vi "Teleop[Conflict].vi"(10 "Match Info":T3={"Autonomous Elapsed Seconds"=0.0, "TeleOp Elapsed Seconds"=0.0, "Disabled Elapsed Seconds"=0.0, "Visited Autonomous"=FALSE, "Visited TeleOp"=FALSE, "Visited Disabled"=FALSE, "Autonomous Settings"={"Autonomous Style"=enum."Independent", "VI Refnum"=refnum}}, 11 "Call Context":T4) -> ()   [LabVIEW 2019]
doc: "This VI is called for each TeleOp packet received from the DS where the robot is not disabled. It is often used to read from the joysticks and update I/O or to update setpoints for timed control loops. It should complete and return within 20 milliseconds or it may miss DS packets."
uses:
  <vilib>/Rock Robotics/WPI/DriverStation/WPI_DriverStationDerivedRobotMode.ctl
  <vilib>/Rock Robotics/WPI/DriverStation/WPI_DriverStationMatch Info.ctl
  <vilib>/Rock Robotics/WPI/ThirdParty/Phoenix-LabVIEW/Motor Controller/Controls/CTRE_Phoenix_MotorControl_ControlMode.ctl
  <vilib>/Rock Robotics/WPI/Utilities/WPI_GetSetVariantRefNum.vi
  <vilib>/Rock Robotics/WPI/Joystick/WPI_JoystickArcadeMapping.vi
  Toolbox/Piston/Piston Toggle.vi
  <vilib>/Rock Robotics/WPI/Solenoid/WPI_SolenoidSetEnum.vi
  <vilib>/Rock Robotics/WPI/ThirdParty/Phoenix-LabVIEW/Motor Controller/Get/CTRE_Phoenix_MotorController_GetSupplyAndStatorCurrent_Enhanced.vi
  <vilib>/Rock Robotics/Network Tables/NT Read Number.vi
  <vilib>/addons/control/pid/pid.llb/PID (DBL).vi
  <vilib>/addons/control/pid/NI_PID_pid.lvlib
panel:
  in  "Shooter Power":dbl=1.0
  in  "Auto Mode":enum16{"Manual", "Old Auto", "New Auto"}(ring)
  in  "Magazine Recovery Power":dbl=0.5
  in  "Magazine Intake power":dbl=0.25
  in  "Idle flywheel power":dbl
  in  "Flywheel power":dbl
  in  "Magazine power":dbl
  in  "Intake power":dbl=0.7
  out "Shooter Motor Current":T1(graph)
  out "tx":dbl
  in  "PID gains":T2={"proportional gain (Kc)"=0.05, "integral time (Ti, min)"=0.0, "derivative time (Td, min)"=0.0} {"derivative time (Td, min)" format="%.3g"; "integral time (Ti, min)" format="%.3e"; "proportional gain (Kc)" format="%.3g"}
  in  "Winch Power":dbl=1.0
  in  "Intake Power":dbl=1.0
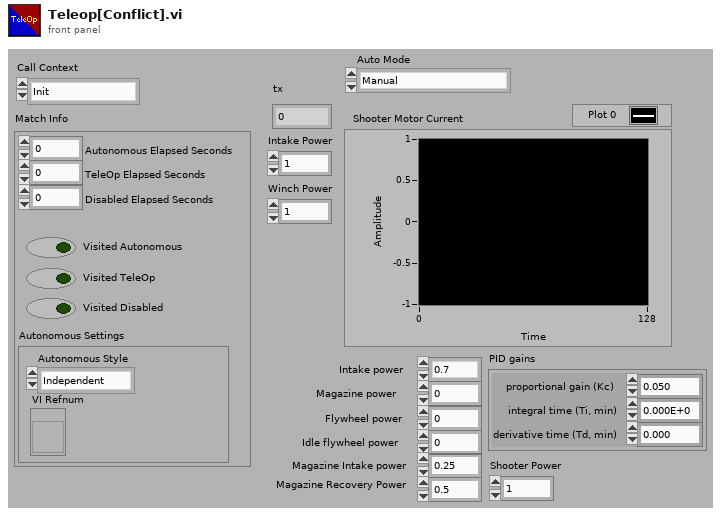
[diagram p1: front panel]
types:
  T1 = cluster{"Supply Current":dbl, "Stator Current":dbl}
  T2 = cluster{"proportional gain (Kc)":dbl, "integral time (Ti, min)":dbl, "derivative time (Td, min)":dbl}
  T3 = typedef "WPI_DriverStationMatch Info.ctl" = cluster{"Autonomous Elapsed Seconds":dbl, "TeleOp Elapsed Seconds":dbl, "Disabled Elapsed Seconds":dbl, "Visited Autonomous":bool, "Visited TeleOp":bool, "Visited Disabled":bool, "Autonomous Settings":cluster{"Autonomous Style":enum16{"Iterative", "Independent"}, "VI Refnum":refnum<vi>}}
  T4 = typedef "WPI_DriverStationDerivedRobotMode.ctl" = enum16{"Init", "Execute", "Stop"}
  T5 = cluster{"Intake In":bool, "Intake Out":bool, "Magazine In":bool, "Magazine Out":bool, "Winch In":bool, "Winch Out":bool, "Climber Hold":bool, "Intake Pistons":bool, "Shooter Hold":bool, "None":bool, "Power Toggle":bool, "Auto Target":bool}
  T6 = typedef "CTRE_Phoenix_MotorControl_ControlMode.ctl" = u16
  T7 = typedef "WPI_JoystickDevRef.ctl" = cluster{"Device":T8}
  T8 = typedef "WPI_JoystickDeviceEnum.ctl" = enum16{"USB 0", "USB 1", "USB 2", "USB 3", "USB 4", "USB 5"}
  T9 = typedef "WPI_SolenoidValue.ctl" = enum16{"Off", "On", "Forward", "Reverse"}
  T10 = typedef "WPI_SolenoidDevRef.ctl" = cluster{"DevStatus":errorcluster, "Pneumatics Control Module":u8, "Forward Solenoid Channel":T11, "Reverse Solenoid Channel":T11}
  T11 = typedef "WPI_SolenoidChannel.ctl" = enum8{"Solenoid 0", "Solenoid 1", "Solenoid 2", "Solenoid 3", "Solenoid 4", "Solenoid 5", "Solenoid 6", "Solenoid 7", "Invalid"}
  T12 = typedef "WPI_DigitalInputDevRef.ctl" = cluster{"DevStatus":errorcluster, "DIO Channel":T13}
  T13 = typedef "FPGA_DIOChannel.ctl" = enum8{"DIO 0", "DIO 1", "DIO 2", "DIO 3", "DIO 4", "DIO 5", "DIO 6", "DIO 7", "DIO 8", "DIO 9", "DIO MXP 0", "DIO MXP 1", "DIO MXP 2", "DIO MXP 3", "DIO MXP 4", "DIO MXP 5", "DIO MXP 6", "DIO MXP 7", "DIO MXP 8", "DIO MXP 9", "DIO MXP 10", "DIO MXP 11", "DIO MXP 12", "DIO MXP 13", "DIO MXP 14", "DIO MXP 15", "SPI Port CS1", "SPI Port CS2", "SPI Port CS3", "SPI Port MISO", "SPI Port MOSI", "Invalid"}
  T14 = typedef "WPI_MotorControlDeviceRef.ctl" = cluster{"DeviceStatus":errorcluster, "Type":T15, "PWM":cluster{"PWM Channel":T16, "DeadBand":T17}, "CAN":cluster{"Device Number":u8, "SetOutput VI Ref":variant, "GetOutput VI Ref":variant, "Enable VI Ref":variant, "Disable VI Ref":variant, "Data":variant}, "Invert":bool, "DIO PWM":cluster{"PWM \"Enable\" Channel":T16, "DIOChannel":T13, "PWM Rate":dbl}}
  T15 = typedef "WPI_MotorControlType.ctl" = enum16{"PWM", "CAN", "DIO PWM"}
  T16 = typedef "FPGA_DIOPWMChannel.ctl" = enum8{"PWM 0", "PWM 1", "PWM 2", "PWM 3", "PWM 4", "PWM 5", "PWM 6", "PWM 7", "PWM 8", "PWM 9", "PWM MXP 0", "PWM MXP 1", "PWM MXP 2", "PWM MXP 3", "PWM MXP 4", "PWM MXP 5", "PWM MXP 6", "PWM MXP 7", "PWM MXP 8", "PWM MXP 9", "Invalid"}
  T17 = typedef "WPI_PWMDeadband.ctl" = cluster{"Name":string, "maxPositivePwm":i32, "minPositivePwm":i32, "centerPwm":i32, "maxNegativePwm":i32, "minNegativePwm":i32, "angularRange":u16}
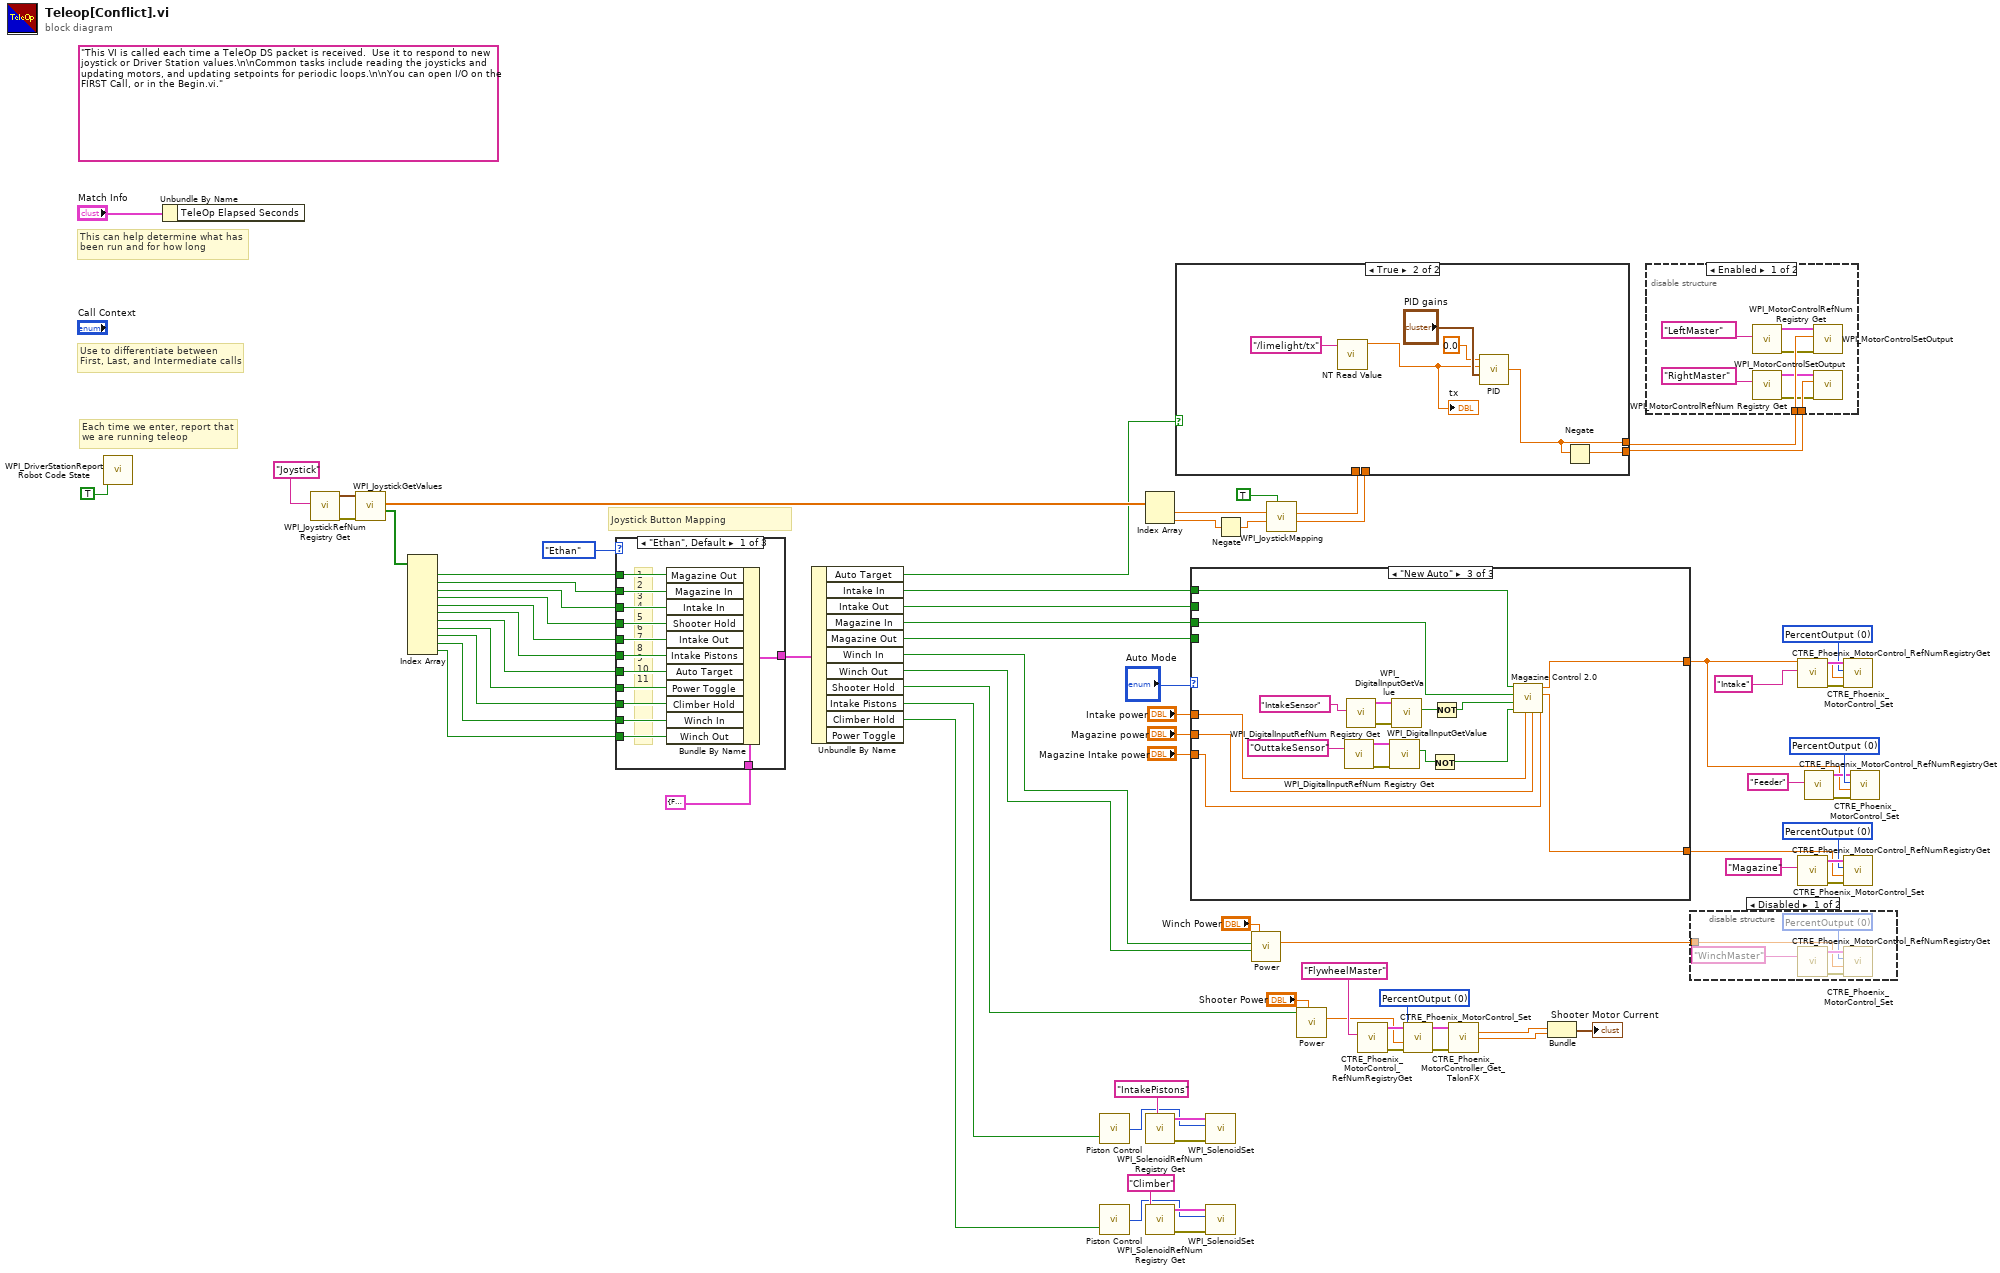
[diagram p0: block diagram]
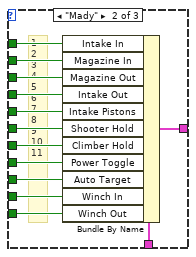
[diagram p2: hidden frame]
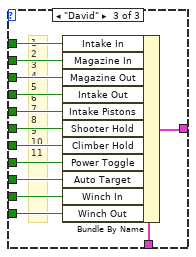
[diagram p3: hidden frame]
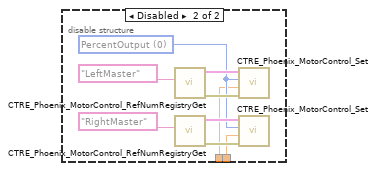
[diagram p5: hidden frame]
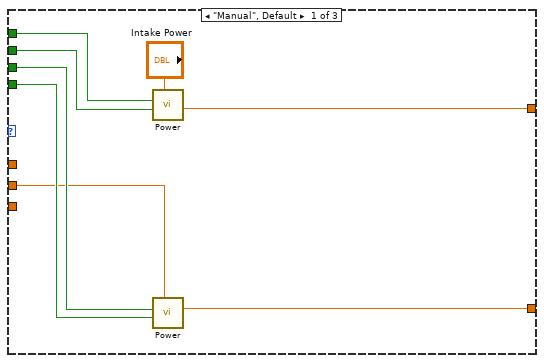
[diagram p7: hidden frame]
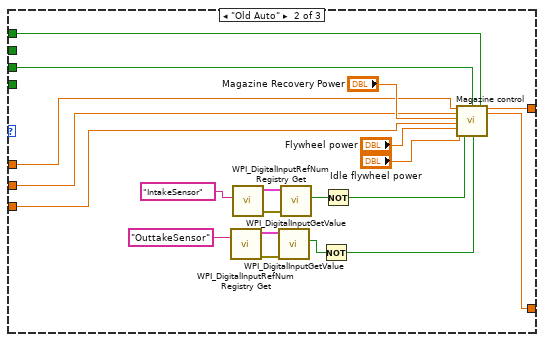
[diagram p8: hidden frame]
diagram:
  w24 = T6 0 items=["PercentOutput"=0, "Position"=1, "Velocity"=2, "Current"=3, "Follower"=5, "MotionProfile"=6, "MotionMagic"=7, "MotionProfileArc"=10, "Disabled"=15] ("Control Mode")
  w57 = T6 0 items=["PercentOutput"=0, "Position"=1, "Velocity"=2, "Current"=3, "Follower"=5, "MotionProfile"=6, "MotionMagic"=7, "MotionProfileArc"=10, "Disabled"=15] ("Control Mode")
  w56 = T6 0 items=["PercentOutput"=0, "Position"=1, "Velocity"=2, "Current"=3, "Follower"=5, "MotionProfile"=6, "MotionMagic"=7, "MotionProfileArc"=10, "Disabled"=15] ("Control Mode")
  w65 = T6 0 items=["PercentOutput"=0, "Position"=1, "Velocity"=2, "Current"=3, "Follower"=5, "MotionProfile"=6, "MotionMagic"=7, "MotionProfileArc"=10, "Disabled"=15] ("Control Mode")
  (unwired) "This VI is called each time a TeleOp DS packet is received.  Use it to respond to new joystick or Driver Station values.\n\nCommon tasks include reading the joysticks and updating motors, and updating setpoints for periodic loops.\n\nYou can open I/O on the FIRST Call, or in the Begin.vi."
  # "Joystick Button Mapping"
  # "Each time we enter, report that\nwe are running teleop"
  # "Use to differentiate between\nFirst, Last, and Intermediate calls"
  # "This can help determine what has\nbeen run and for how long"
  n1 = call <vilib>:"WPI_DriverStationReport Robot Code State.vi"("TeleOp"=TRUE ("Autonomous")) -> ()  [unwired: 10 in, 1 out]
  n2 = Unbundle By Name("Match Info") -> ()  [unwired: 1 out]
  n3 = call <vilib>:"WPI_JoystickRefNum Registry Get.vi"("refnum name"="Joystick") -> ("error out"=w76:errorcluster, "JoystickDevRef"=w75:T7)  [unwired: 9 in]
  n4 = call <vilib>:"WPI_JoystickGetValues.vi"("error in (no error)"=w76, "JoystickDevRef"=w75) -> ("Buttons"=w46:bool[], "Axes"=w73:dbl[])  [unwired: 5 in, 3 out]
  n5 = Index Array(array=w46) -> (element #1=w47:bool, element #2=w1:bool, element #3=w55:bool, element #4=w2:bool, element #5=w54:bool, element #6=w53:bool, element #7=w52:bool, element #8=w51:bool, element #9=w50:bool, element #10=w49:bool, element #11=w48:bool)  [unwired: 11 in]
  n6 = case shown="\"Ethan\", Default" enum16{"Ethan", "Mady", "David"}."Ethan" {
    tunnel: w1 -> [w90 w104 w106]
    tunnel: w55 -> [w89 w103 w107]
    tunnel: w2 -> [w88 w102 w108]
    tunnel: w54 -> [w87 w101 w109]
    tunnel: w53 -> [w86 w100 w110]
    tunnel: w52 -> [w85 w99 w111]
    tunnel: w51 -> [w84 w98 w112]
    tunnel: w50 -> [w83 w97 w113]
    tunnel: w49 -> [w82 w96 w114]
    tunnel: w48 -> [w81 w95 w115]
    tunnel: w47 -> [w91 w94 w105]
    tunnel: [w80 w93 w117] -> w45
    tunnel: T5 {"Intake In"=FALSE, "Intake Out"=FALSE, "Magazine In"=FALSE, "Magazine Out"=FALSE, "Winch In"=FALSE, "Winch Out"=FALSE, "Climber Hold"=FALSE, "Intake Pistons"=FALSE, "Shooter Hold"=FALSE, "None"=FALSE, "Power Toggle"=FALSE, "Auto Target"=FALSE} ("input cluster") -> [w79 w92 w116]
    frame "Ethan", Default {
      # "1\n2\n3\n4\n5\n6\n7\n8\n9\n10\n11"
      n7 = Bundle By Name(cluster=w79, "Magazine Out"=w91, "Magazine In"=w90, "Intake In"=w89, "Shooter Hold"=w88, "Intake Out"=w87, "Intake Pistons"=w86, "Auto Target"=w85, "Power Toggle"=w84, "Climber Hold"=w83, "Winch In"=w82, "Winch Out"=w81) -> (w80:T5)
    }
    frame "Mady" {
      # "1\n2\n3\n4\n5\n6\n7\n8\n9\n10\n11"
      n8 = Bundle By Name(cluster=w92, "Intake In"=w94, "Magazine In"=w104, "Magazine Out"=w103, "Intake Out"=w102, "Intake Pistons"=w101, "Shooter Hold"=w100, "Climber Hold"=w99, "Power Toggle"=w98, "Auto Target"=w97, "Winch In"=w96, "Winch Out"=w95) -> (w93:T5)
    }
    frame "David" {
      # "1\n2\n3\n4\n5\n6\n7\n8\n9\n10\n11"
      n9 = Bundle By Name(cluster=w116, "Intake In"=w105, "Magazine In"=w106, "Magazine Out"=w107, "Intake Out"=w108, "Intake Pistons"=w109, "Shooter Hold"=w110, "Climber Hold"=w111, "Power Toggle"=w112, "Auto Target"=w113, "Winch In"=w114, "Winch Out"=w115) -> (w117:T5)
    }
  }
  n10 = Unbundle By Name(w45) -> ("Auto Target"=w14:bool, "Intake In"=w27:bool, "Intake Out"=w44:bool, "Magazine In"=w43:bool, "Magazine Out"=w42:bool, "Winch In"=w41:bool, "Winch Out"=w40:bool, "Shooter Hold"=w28:bool, "Intake Pistons"=w11:bool, "Climber Hold"=w10:bool)  [unwired: 1 out]
  n11 = call-poly "Piston Control.vi"("Input"=w11) -> ("Output"=w13:T9)  [unwired: 1 in]
  n12 = call-poly "Piston Control.vi"("Input"=w10) -> ("Output"=w12:T9)  [unwired: 1 in]
  n13 = Index Array(array=w73) -> (element #1=w72:dbl, element #2=w70:dbl)  [unwired: 2 in]
  n14 = call <vilib>:"WPI_SolenoidRefNum Registry Get.vi"("refnum name"="IntakePistons") -> ("error out"=w39:errorcluster, "SolenoidDevRef"=w38:T10)  [unwired: 9 in]
  n15 = call <vilib>:"WPI_SolenoidRefNum Registry Get.vi"("refnum name"="Climber") -> ("error out"=w36:errorcluster, "SolenoidDevRef"=w35:T10)  [unwired: 9 in]
  n16 = case shown="\"New Auto\"" "Auto Mode" {
    tunnel: w44 -> [w125 _ _]
    tunnel: w43 -> [w124 w129 w151]
    tunnel: w42 -> [w123 _ _]
    tunnel: w27 -> [w122 w130 w152]
    tunnel: [w119 w137 w150] -> w19
    tunnel: [w120 w136 w149] -> w20
    tunnel: "Magazine Intake power" -> [_ w128 w146]
    tunnel: "Magazine power" -> [w118 w127 w147]
    tunnel: "Intake power" -> [_ w126 w148]
    frame "Manual", Default {
      n17 = call "Power.vi"("Positive Power"="Intake Power", "Negative"=w125, "Positive"=w122) -> ("Output"=w119:dbl)  [unwired: 8 in]
      n18 = call "Power.vi"("Positive Power"=w118, "Negative"=w123, "Positive"=w124) -> ("Output"=w120:dbl)  [unwired: 8 in]
    }
    frame "Old Auto" {
      n19 = call <vilib>:"WPI_DigitalInputRefNum Registry Get.vi"("refnum name"="OuttakeSensor") -> ("error out"=w143:errorcluster, "DigitalInputDevRef"=w142:T12)  [unwired: 9 in]
      n20 = call <vilib>:"WPI_DigitalInputRefNum Registry Get.vi"("refnum name"="IntakeSensor") -> ("error out"=w140:errorcluster, "DigitalInputDevRef"=w141:T12)  [unwired: 9 in]
      n21 = call <vilib>:"WPI_DigitalInputGetValue.vi"("error in (no error)"=w143, "DigitalInputDevRef"=w142) -> ("Value"=w145:bool)  [unwired: 7 in, 2 out]
      n22 = call <vilib>:"WPI_DigitalInputGetValue.vi"("error in (no error)"=w140, "DigitalInputDevRef"=w141) -> ("Value"=w144:bool)  [unwired: 7 in, 2 out]
      n23 = Not(x=w145) -> (.not. x?=w135:bool)
      n24 = Not(x=w144) -> (.not. x?=w134:bool)
      n25 = call "Magazine control.vi"("Intake power"=w126, "Magazine power"=w127, "Magazine Recovery Power"="Magazine Recovery Power", "Magazine Intake power"=w128, "Flywheel power"="Flywheel power", "Idle flywheel power"="Idle flywheel power", "Intake sensor"=w134, "Intake"=w130, "Shoot"=w129, "Outtake sensor"=w135) -> ("Intake"=w137:dbl, "Magazine"=w136:dbl)  [unwired: 7 in, 1 out]
    }
    frame "New Auto" {
      n26 = call <vilib>:"WPI_DigitalInputRefNum Registry Get.vi"("refnum name"="OuttakeSensor") -> ("error out"=w159:errorcluster, "DigitalInputDevRef"=w160:T12)  [unwired: 9 in]
      n27 = call <vilib>:"WPI_DigitalInputRefNum Registry Get.vi"("refnum name"="IntakeSensor") -> ("error out"=w162:errorcluster, "DigitalInputDevRef"=w161:T12)  [unwired: 9 in]
      n28 = call <vilib>:"WPI_DigitalInputGetValue.vi"("error in (no error)"=w159, "DigitalInputDevRef"=w160) -> ("Value"=w157:bool)  [unwired: 7 in, 2 out]
      n29 = call <vilib>:"WPI_DigitalInputGetValue.vi"("error in (no error)"=w162, "DigitalInputDevRef"=w161) -> ("Value"=w158:bool)  [unwired: 7 in, 2 out]
      n30 = Not(x=w157) -> (.not. x?=w153:bool)
      n31 = Not(x=w158) -> (.not. x?=w154:bool)
      n32 = call "Magazine Control 2.0.vi"("Magazine Overflow Power"=w146, "Magazine Power"=w147, "Intake Power"=w148, "Outtake Sensor"=w153, "Intake Sensor"=w154, "Outtake Button"=w151, "Intake Button"=w152) -> ("Magazine"=w149:dbl, "Intake"=w150:dbl)  [unwired: 3 in]
    }
  }
  n33 = call-poly <vilib>:"WPI_SolenoidSet.vi"("error in (no error)"=w39, "Value"=w13, "SolenoidDevRef"=w38) -> ()  [unwired: 7 in, 2 out]
  n34 = call-poly <vilib>:"WPI_SolenoidSet.vi"("error in (no error)"=w36, "Value"=w12, "SolenoidDevRef"=w35) -> ()  [unwired: 7 in, 2 out]
  n35 = Negate(x=w70) -> (-x=w71:dbl)
  n36 = call "Power.vi"("Positive Power"="Winch Power", "Negative"=w40, "Positive"=w41) -> ("Output"=w61:dbl)  [unwired: 8 in]
  n37 = call-poly <vilib>:"WPI_JoystickMapping.vi"("Square Inputs"=TRUE, "Y axis value"=w71, "X axis value"=w72) -> ("Right Motor Value"=w17:dbl, "Left Motor Value"=w18:dbl)  [unwired: 7 in]
  n38 = case shown="True" w14 {
    tunnel: w18 -> [w164 _]
    tunnel: w17 -> [w163 _]
    tunnel: [w164 w165] -> w16
    tunnel: [w163 w166] -> w15
    frame False {
    }
    frame True {
      n39 = call-poly <vilib>:"NT Read Value.vi"("Name"="/limelight/tx") -> ("Numeric"=w169:dbl)  [unwired: 9 in, 1 out]
      "tx" <- w169
      n40 = call-poly <vilib>:"PID.vi"("PID gains"="PID gains", "process variable"=w169, "setpoint"=0.0) -> ("output"=w165:dbl)  [unwired: 7 in, 1 out]
      n41 = Negate(x=w165) -> (-x=w166:dbl)
    }
  }
  n42 = call "Power.vi"("Positive Power"="Shooter Power", "Positive"=w28) -> ("Output"=w25:dbl)  [unwired: 9 in]
  n43 = call <vilib>:"CTRE_Phoenix_MotorControl_RefNumRegistryGet.vi"("refnum name"="FlywheelMaster") -> ("error out"=w59:errorcluster, "PhoenixMotorControlDevRef"=w58:T14)  [unwired: 9 in]
  n44 = call <vilib>:"CTRE_Phoenix_MotorControl_Set.vi"("error in (no error)"=w59, "Output"=w25, "Control Mode"=w57, "PhoenixMotorControlDevRef"=w58) -> ("error out"=w32:errorcluster, "PhoenixMotorControlDevRef"=w33:T14)  [unwired: 6 in]
  n45 = call-poly <vilib>:"CTRE_Phoenix_MotorController_Get_TalonFX.vi"("PhoenixMotorControlDevRef"=w33, "error in"=w32) -> ("Supply Current"=w31:dbl, "Stator Current"=w30:dbl)  [unwired: 10 in, 2 out]
  n46 = Bundle("Supply Current"=w31, "Stator Current"=w30) -> (→"Shooter Motor Current":T1)  [unwired: 1 in]
  n47 = disable-structure shown="Enabled" {
    disable-tunnel: w16 -> [w178 w180]
    disable-tunnel: w15 -> [w177 w179]
    frame Enabled {
      n48 = call <vilib>:"WPI_MotorControlRefNum Registry Get.vi"("refnum name"="LeftMaster") -> ("error out"=w174:errorcluster, "MotorControlDevRef"=w173:T14)  [unwired: 9 in]
      n49 = call <vilib>:"WPI_MotorControlRefNum Registry Get.vi"("refnum name"="RightMaster") -> ("error out"=w172:errorcluster, "MotorControlDevRef"=w171:T14)  [unwired: 9 in]
      n50 = call <vilib>:"WPI_MotorControlSetOutput.vi"("error in (no error)"=w174, "Output"=w178, "MotorControlDevRef"=w173) -> ()  [unwired: 6 in, 3 out]
      n51 = call <vilib>:"WPI_MotorControlSetOutput.vi"("error in (no error)"=w172, "Output"=w177, "MotorControlDevRef"=w171) -> ()  [unwired: 6 in, 3 out]
    }
    frame Disabled {
      w181 = T6 0 items=["PercentOutput"=0, "Position"=1, "Velocity"=2, "Current"=3, "Follower"=5, "MotionProfile"=6, "MotionMagic"=7, "MotionProfileArc"=10, "Disabled"=15] ("Control Mode")
      n52 = call <vilib>:"CTRE_Phoenix_MotorControl_RefNumRegistryGet.vi"("refnum name"="LeftMaster") -> ("error out"=w185:errorcluster, "PhoenixMotorControlDevRef"=w184:T14)  [unwired: 9 in]
      n53 = call <vilib>:"CTRE_Phoenix_MotorControl_RefNumRegistryGet.vi"("refnum name"="RightMaster") -> ("error out"=w183:errorcluster, "PhoenixMotorControlDevRef"=w182:T14)  [unwired: 9 in]
      n54 = call <vilib>:"CTRE_Phoenix_MotorControl_Set.vi"("error in (no error)"=w185, "Output"=w180, "Control Mode"=w181, "PhoenixMotorControlDevRef"=w184) -> ()  [unwired: 6 in, 2 out]
      n55 = call <vilib>:"CTRE_Phoenix_MotorControl_Set.vi"("error in (no error)"=w183, "Output"=w179, "Control Mode"=w181, "PhoenixMotorControlDevRef"=w182) -> ()  [unwired: 6 in, 2 out]
    }
  }
  n56 = disable-structure shown="Disabled" {
    disable-tunnel: w61 -> [w188 _]
    frame Disabled {
      w189 = T6 0 items=["PercentOutput"=0, "Position"=1, "Velocity"=2, "Current"=3, "Follower"=5, "MotionProfile"=6, "MotionMagic"=7, "MotionProfileArc"=10, "Disabled"=15] ("Control Mode")
      n57 = call <vilib>:"CTRE_Phoenix_MotorControl_RefNumRegistryGet.vi"("refnum name"="WinchMaster") -> ("error out"=w191:errorcluster, "PhoenixMotorControlDevRef"=w190:T14)  [unwired: 9 in]
      n58 = call <vilib>:"CTRE_Phoenix_MotorControl_Set.vi"("error in (no error)"=w191, "Output"=w188, "Control Mode"=w189, "PhoenixMotorControlDevRef"=w190) -> ()  [unwired: 6 in, 2 out]
    }
    frame Enabled {
    }
  }
  n59 = call <vilib>:"CTRE_Phoenix_MotorControl_RefNumRegistryGet.vi"("refnum name"="Intake") -> ("error out"=w63:errorcluster, "PhoenixMotorControlDevRef"=w64:T14)  [unwired: 9 in]
  n60 = call <vilib>:"CTRE_Phoenix_MotorControl_RefNumRegistryGet.vi"("refnum name"="Magazine") -> ("error out"=w67:errorcluster, "PhoenixMotorControlDevRef"=w66:T14)  [unwired: 9 in]
  n61 = call <vilib>:"CTRE_Phoenix_MotorControl_RefNumRegistryGet.vi"("refnum name"="Feeder") -> ("error out"=w22:errorcluster, "PhoenixMotorControlDevRef"=w23:T14)  [unwired: 9 in]
  n62 = call <vilib>:"CTRE_Phoenix_MotorControl_Set.vi"("error in (no error)"=w63, "Output"=w19, "Control Mode"=w56, "PhoenixMotorControlDevRef"=w64) -> ()  [unwired: 6 in, 2 out]
  n63 = call <vilib>:"CTRE_Phoenix_MotorControl_Set.vi"("error in (no error)"=w67, "Output"=w20, "Control Mode"=w65, "PhoenixMotorControlDevRef"=w66) -> ()  [unwired: 6 in, 2 out]
  n64 = call <vilib>:"CTRE_Phoenix_MotorControl_Set.vi"("error in (no error)"=w22, "Output"=w19, "Control Mode"=w24, "PhoenixMotorControlDevRef"=w23) -> ()  [unwired: 6 in, 2 out]
